vi "main.vi"() -> ()   [LabVIEW 2014]
doc: "为该项目的启动vi"
uses:
  R/manifest.vi
  glb/glb_static.vi
panel:
  in  "Player":refnum<k7>(container)
  in  "停止":bool
  in  "视屏1":bool
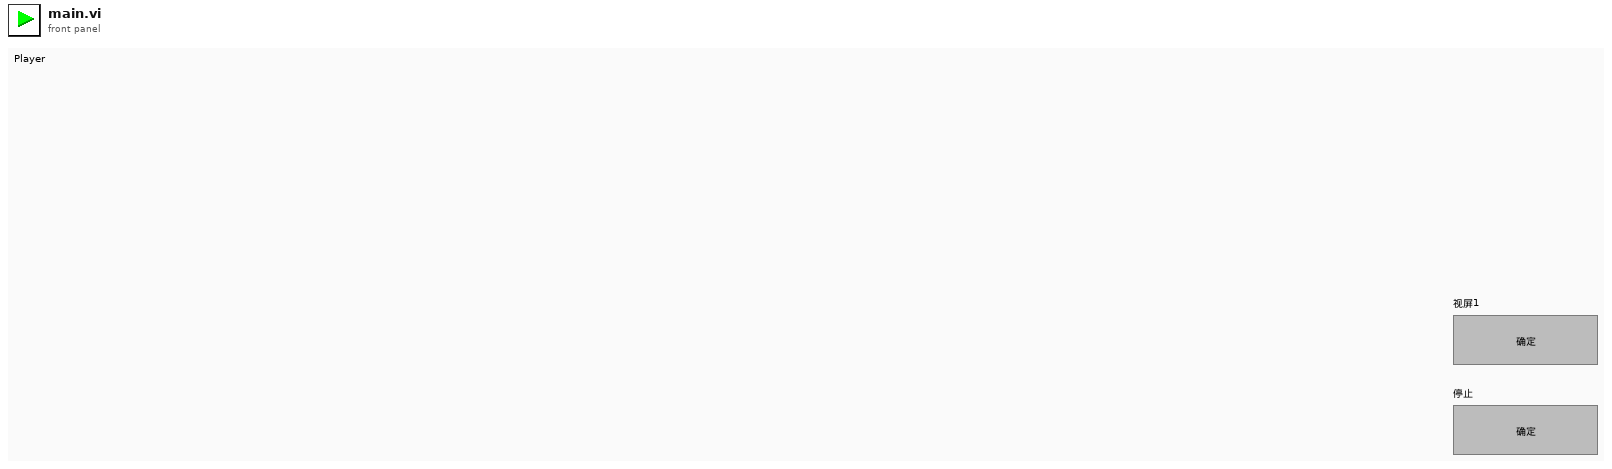
[diagram p1: front panel]
types:
  T1 = cluster{"标题":string, "相对路径":string, "类型":enum16{"服务", "活动"}, "专属队列名称":string}
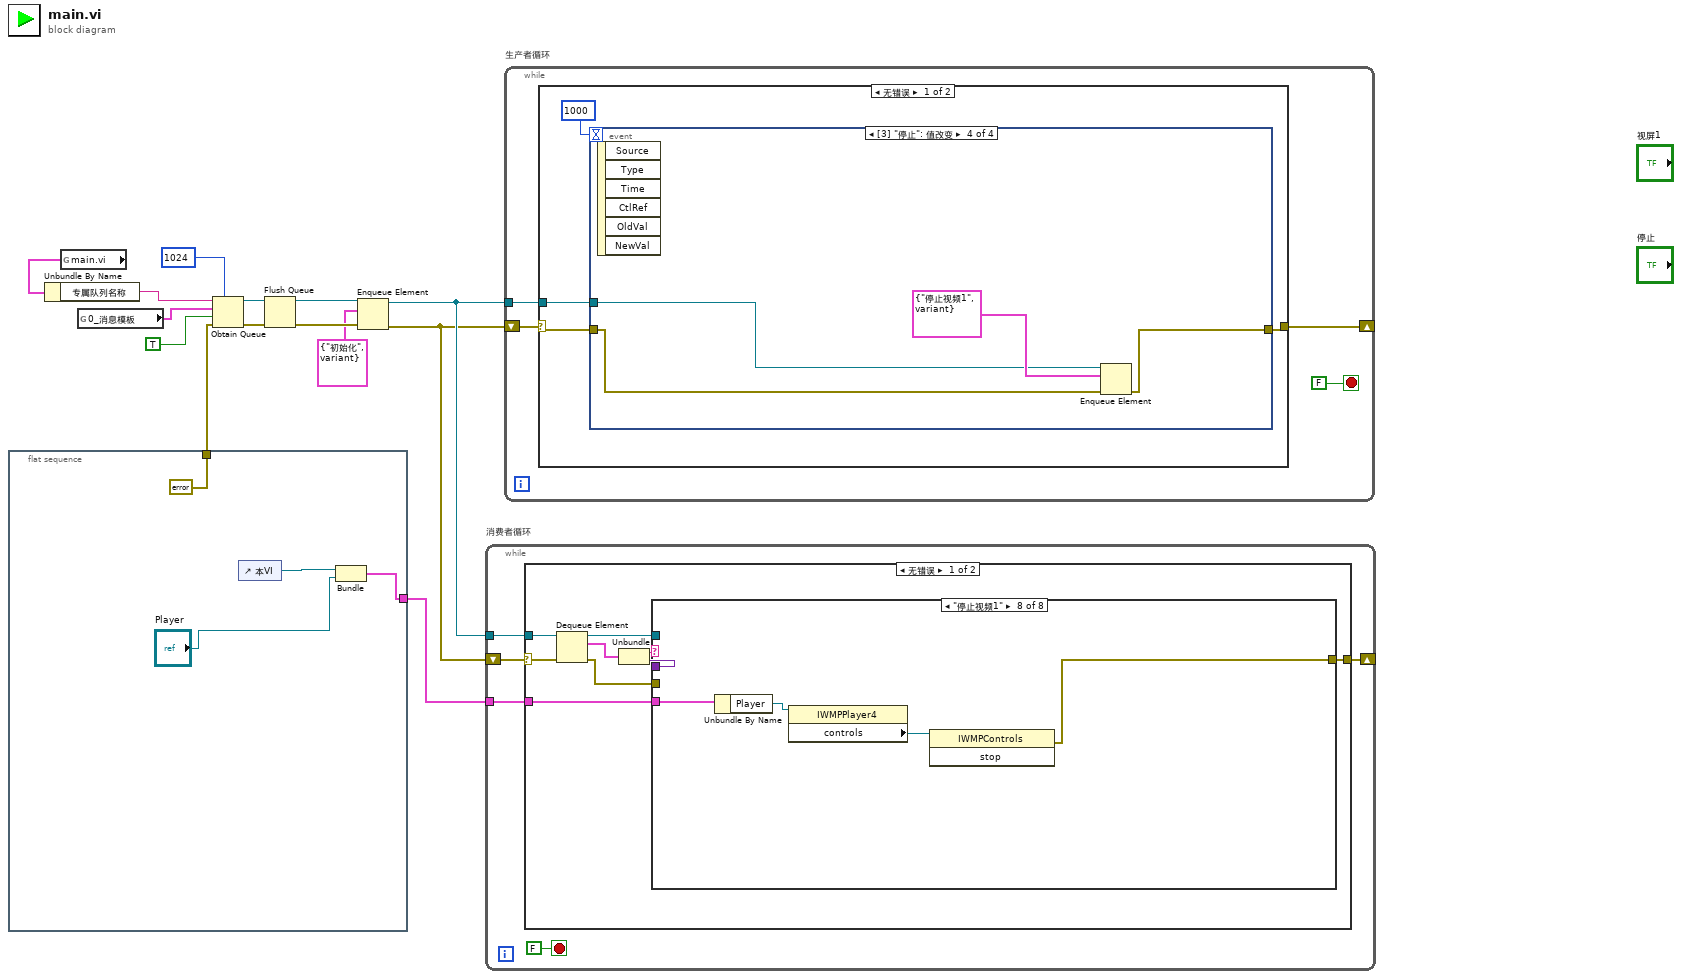
[diagram p0: block diagram]
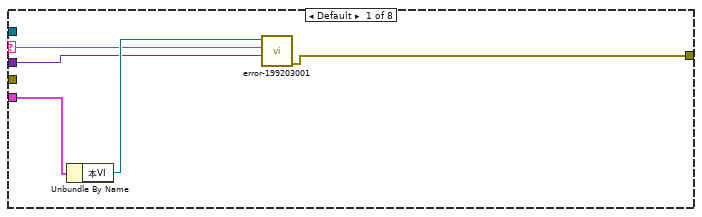
[diagram p2: hidden frame]
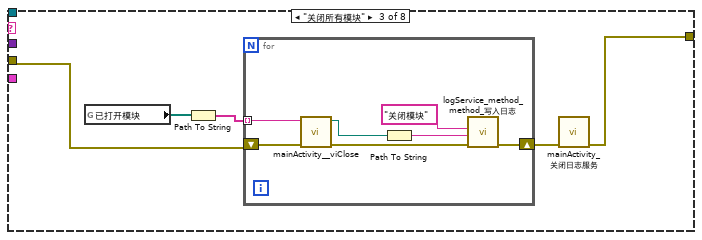
[diagram p4: hidden frame]
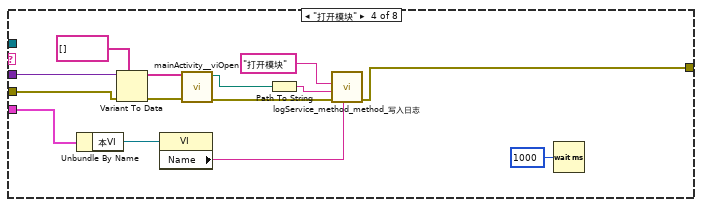
[diagram p5: hidden frame]
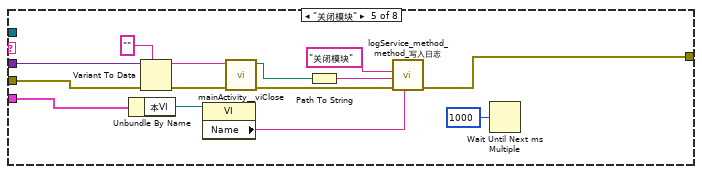
[diagram p6: hidden frame]
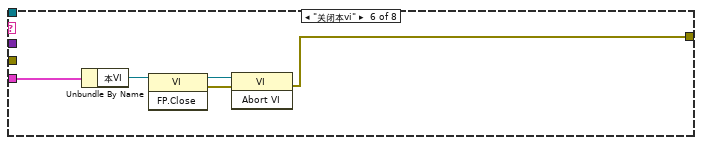
[diagram p7: hidden frame]
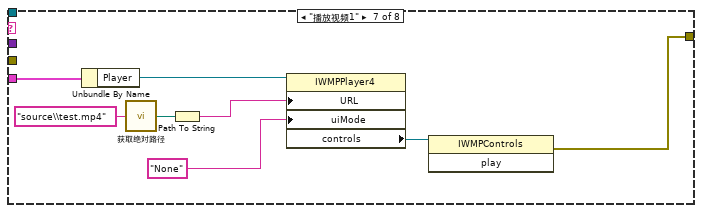
[diagram p8: hidden frame]
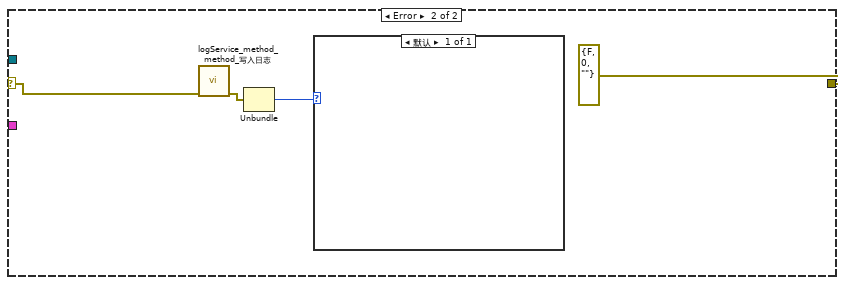
[diagram p9: hidden frame]
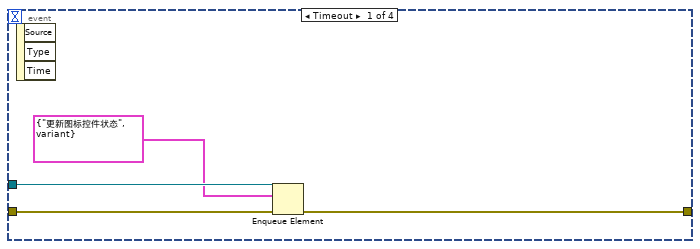
[diagram p10: hidden frame]
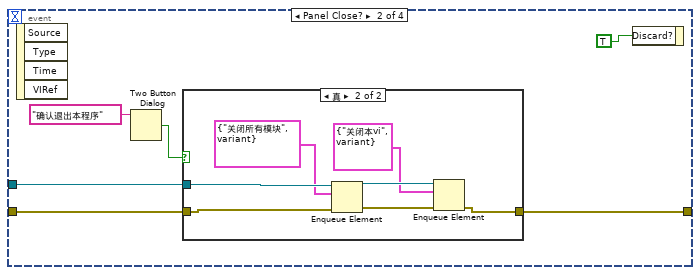
[diagram p11: hidden frame]
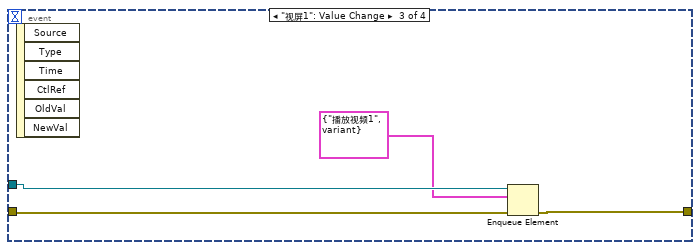
[diagram p13: hidden frame]
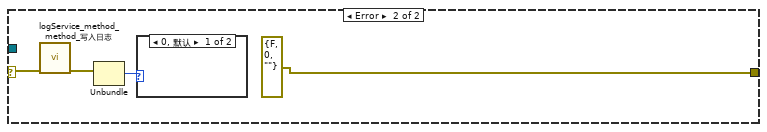
[diagram p14: hidden frame]
diagram:
  n1 = flat-sequence {
    tunnel: [errorcluster {"status"=FALSE, "code"=0, "source"=""} ("error out")] -> w1
    tunnel: [w16] -> w2
    frame #0 {
      n2 = control-ref of="本VI"() -> (w17:refnum<vi>)
      n3 = Bundle("本VI"=w17, "Player"="Player") -> (w16:cluster{"本VI":refnum<vi>, "Player":refnum<k7>})  [unwired: 1 in]
    }
  }
  n4 = global read "manifest.vi" "main.vi"() -> (w9:T1)
  n5 = Unbundle By Name(w9) -> ("专属队列名称"=w8:string)
  n6 = global read "manifest.vi" "0_消息模板"() -> (w7:cluster{"消息":string, "数据":variant})
  n7 = Obtain Queue(max queue size (-1, unlimited)=1024 ("队列最大值（-1，无限）"), name (unnamed)=w8, element data type=w7, create if not found? (T)=TRUE ("如未找到是否创建？(T)"), error in (no error)=w1) -> (queue out=w3:refnum<queue>, error out=w4:errorcluster)  [unwired: 1 out]
  n8 = Flush Queue(queue=w3, error in (no error)=w4) -> (queue out=w14:refnum<queue>, error out=w12:errorcluster)  [unwired: 1 out]
  n9 = Enqueue Element(queue=w14, element=cluster{"message":string, "data":variant} {"message"="初始化", "data"=variant} ("元素"), error in (no error)=w12) -> (queue out=w13:refnum<queue>, error out=w11:errorcluster)  [unwired: 1 in, 1 out]
  n10 = while "消费者循环" {
    tunnel: w13 -> [w22]
    shift-right: [w21] -> _
    shift-left: w11 -> [w23]
    tunnel: w2 -> [w20]
    stop <- FALSE stop-if-true
    n11 = case shown="无错误" w23 {
      selector: w23 -> [w31 w98]
      tunnel: w22 -> [w32 _]
      tunnel: [w25 errorcluster {"status"=FALSE, "code"=0, "source"=""} ("错误输出")] -> w21
      tunnel: w20 -> [w24 _]
      frame No Error {
        n12 = Dequeue Element(queue=w32, error in (no error)=w31) -> (queue out=w26:refnum<queue>, element=w30:cluster{"消息":string, "数据":variant}, error out=w27:errorcluster)  [unwired: 1 in, 1 out]
        n13 = Unbundle(w30) -> ("消息"=w29:string, "数据"=w28:variant)
        n14 = case shown="\"停止视频1\"" w29 {
          selector: w29 -> [w35 _ _ _ _ _ _ _]
          tunnel: w28 -> [w34 _ _ w63 w77 _ _ _]
          tunnel: w27 -> [_ _ w42 w62 w76 _ _ _]
          tunnel: w26 -> [_ _ _ _ _ _ _ _]
          tunnel: [w33 _ w39 w54 w71 w78 w83 w91] -> w25
          tunnel: w24 -> [w37 _ _ w53 w67 w80 w90 w94]
          frame Default {
            n15 = Unbundle By Name(w37) -> ("本VI"=w36:refnum<vi>)
            n16 = call "error-199203001.vi"("数据"=w34, "字符串"=w35, "VI输入"=w36) -> ("错误输出"=w33:errorcluster)  [unwired: 8 in]
          }
          frame "初始化" {
          }
          frame "关闭所有模块" {
            n17 = global read "glb_static.vi" "已打开模块"() -> (w38:path[])
            n18 = Path To String(path=w38) -> (string=w41:string[])
            n19 = for {
              tunnel: w41 -> [w45] mode=indexing
              shift-right: [w43] -> w40
              shift-left: w42 -> [w44]
              n20 = call "mainActivity__viClose.vi"("error in"=w44, "urlStr"=w45) -> ("error out"=w49:errorcluster, "viPath"=w47:path)  [unwired: 8 in]
              n21 = Path To String(path=w47) -> (string=w46:string)
              n22 = call "logService_method_method_写入日志.vi"("error in"=w49, "内容"=w46, "标题"="关闭模块") -> ("error out"=w43:errorcluster)  [unwired: 8 in]
            }
            n23 = call "mainActivity_关闭日志服务.vi"("错误输入（无错误）"=w40) -> ("错误输出"=w39:errorcluster)  [unwired: 10 in]
          }
          frame "打开模块" {
            n24 = Unbundle By Name(w53) -> ("本VI"=w52:refnum<vi>)
            n25 = Variant To Data(error in=w62, type=string[] [], Variant=w63) -> (data=w60:string[], error out=w59:errorcluster)
            n26 = property class="VI"(reference=w52) -> ("Name"=w51:string)  [unwired: 1 in, 2 out]
            n27 = call "mainActivity__viOpen.vi"("error in"=w59, "数组"=w60) -> ("error out"=w58:errorcluster, "viPath"=w56:path)  [unwired: 8 in]
            n28 = Path To String(path=w56) -> (string=w55:string)
            n29 = call "logService_method_method_写入日志.vi"("发生的所在的vi"=w51, "error in"=w58, "内容"=w55, "标题"="打开模块" ("tag")) -> ("error out"=w54:errorcluster)  [unwired: 7 in]
            n30 = Wait (ms)(milliseconds to wait=u32 1000 ("等待时间（毫秒）")) -> ()  [unwired: 1 out]
          }
          frame "关闭模块" {
            n31 = Unbundle By Name(w67) -> ("本VI"=w66:refnum<vi>)
            n32 = Variant To Data(error in=w76, type="", Variant=w77) -> (data=w74:string, error out=w73:errorcluster)
            n33 = property class="VI"(reference=w66) -> ("Name"=w65:string)  [unwired: 1 in, 2 out]
            n34 = call "mainActivity__viClose.vi"("error in"=w73, "urlStr"=w74) -> ("error out"=w72:errorcluster, "viPath"=w69:path)  [unwired: 8 in]
            n35 = Path To String(path=w69) -> (string=w68:string)
            n36 = call "logService_method_method_写入日志.vi"("发生的所在的vi"=w65, "error in"=w72, "内容"=w68, "标题"="关闭模块") -> ("error out"=w71:errorcluster)  [unwired: 7 in]
            n37 = Wait Until Next ms Multiple(millisecond multiple=u32 1000 ("毫秒倍数")) -> ()  [unwired: 1 out]
          }
          frame "关闭本vi" {
            n38 = Unbundle By Name(w80) -> ("本VI"=w79:refnum<vi>)
            n39 = invoke class="VI" method="FP.Close"(reference=w79) -> (reference out=w82:refnum<vi>, error out=w81:errorcluster)  [unwired: 2 in, 1 out]
            n40 = invoke class="VI" method="Abort VI"(reference=w82, error in=w81) -> (error out=w78:errorcluster)  [unwired: 1 in, 2 out]
          }
          frame "播放视频1" {
            n41 = Unbundle By Name(w90) -> ("Player"=w89:refnum<k7>)
            n42 = call "获取绝对路径.vi"("relativePath"="source\\test.mp4") -> ("absolutePath"=w86:path)
            n43 = Path To String(path=w86) -> (string=w85:string)
            n44 = property class="IWMPPlayer4"(reference=w89, "URL"=w85, "uiMode"="None") -> ("controls"=w84:refnum<k7>)  [unwired: 1 in, 2 out]
            n45 = invoke class="IWMPControls" method="play"(reference=w84) -> (error out=w83:errorcluster)  [unwired: 2 in, 2 out]
          }
          frame "停止视频1" {
            n46 = Unbundle By Name(w94) -> ("Player"=w93:refnum<k7>)
            n47 = property class="IWMPPlayer4"(reference=w93) -> ("controls"=w92:refnum<k7>)  [unwired: 1 in, 2 out]
            n48 = invoke class="IWMPControls" method="stop"(reference=w92) -> (error out=w91:errorcluster)  [unwired: 2 in, 2 out]
          }
        }
      }
      frame Error {
        n49 = call "logService_method_method_写入日志.vi"("error in"=w98) -> ("error out"=w97:errorcluster)  [unwired: 10 in]
        n50 = Unbundle(w97) -> ("code"=w96:i32)  [unwired: 2 out]
        n51 = case shown="默认" w96 {
          frame 默认 {
          }
        }
      }
    }
  }
  n52 = while "生产者循环" {
    tunnel: w13 -> [w101]
    shift-right: [w100] -> _
    shift-left: w11 -> [w102]
    stop <- FALSE stop-if-true
    n53 = case shown="无错误" w102 {
      selector: w102 -> [w105 w136]
      tunnel: w101 -> [w104 _]
      tunnel: [w106 errorcluster {"status"=FALSE, "code"=0, "source"=""} ("error out")] -> w100
      frame No Error {
        n54 = event shown="[3] \"停止\": 值改变" {
          selector: _ -> [_ _ _ _]
          dyn-events: _ -> [_ _ _ _]
          timeout: 1000 -> [_ _ _ _]
          tunnel: [w110 w112 w128 w129] -> w106
          tunnel: w105 -> [w109 w114 w127 w130]
          tunnel: w104 -> [w108 w113 w126 w131]
          event Timeout {
            n55 = event-data() -> ()  [unwired: 1 in, 3 out]
            n56 = Enqueue Element(queue=w108, element=cluster{"message":string, "data":variant} {"message"="更新图标控件状态", "data"=variant} ("元素"), error in (no error)=w109) -> (error out=w110:errorcluster)  [unwired: 1 in, 2 out]
          }
          event Panel Close? {
            n57 = event-data() -> ()  [unwired: 1 in, 4 out]
            n58 = Two Button Dialog(message="确认退出本程序" ("消息")) -> (T button?=w115:bool)  [unwired: 2 in]
            n59 = case shown="真" w115 {
              tunnel: w114 -> [w117 w124]
              tunnel: w113 -> [_ w123]
              tunnel: [w117 w120] -> w112
              frame False {
              }
              frame True {
                n60 = Enqueue Element(queue=w123, element=cluster{"message":string, "data":variant} {"message"="关闭所有模块", "data"=variant} ("元素"), error in (no error)=w124) -> (queue out=w119:refnum<queue>, error out=w121:errorcluster)  [unwired: 1 in, 1 out]
                n61 = Enqueue Element(queue=w119, element=cluster{"message":string, "data":variant} {"message"="关闭本vi", "data"=variant} ("元素"), error in (no error)=w121) -> (error out=w120:errorcluster)  [unwired: 1 in, 2 out]
              }
            }
            n62 = event-data("Discard?"=TRUE) -> ()  [unwired: 1 in, 1 out]
          }
          event "视屏1": Value Change {
            n63 = event-data() -> ()  [unwired: 1 in, 6 out]
            n64 = Enqueue Element(queue=w126, element=cluster{"消息":string, "数据":variant} {"消息"="播放视频1", "数据"=variant} ("元素"), error in (no error)=w127) -> (error out=w128:errorcluster)  [unwired: 1 in, 2 out]
          }
          event "停止": Value Change {
            n65 = event-data() -> ()  [unwired: 1 in, 6 out]
            n66 = Enqueue Element(queue=w131, element=cluster{"消息":string, "数据":variant} {"消息"="停止视频1", "数据"=variant} ("元素"), error in (no error)=w130) -> (error out=w129:errorcluster)  [unwired: 1 in, 2 out]
          }
        }
      }
      frame Error {
        n67 = call "logService_method_method_写入日志.vi"("error in"=w136) -> ("error out"=w135:errorcluster)  [unwired: 10 in]
        n68 = Unbundle(w135) -> ("code"=w134:i32)  [unwired: 2 out]
        n69 = case shown="0, 默认" w134 {
          frame 0, Default {
          }
          frame 1 {
          }
        }
      }
    }
  }
